vi "State_Machine.vi"(8 "error in (no error)":errorcluster caption="entrée d'erreur (pas d'erreur)", 11 "Get_Voltage en entrée":refnum<class "Enable_Power_Supply.lvclass">) -> (0 "error out":errorcluster caption="sortie d'erreur", 2 "Json_String":string, 3 "Get_Voltage en sortie":refnum<class "Enable_Power_Supply.lvclass">)   [LabVIEW 2020, in "Library Test.lvlib" / "Enable_Power_Supply.lvclass"]
uses:
  Enable_Power_Supply.lvclass
  C:/Users/ngarcin/OneDrive - Altyor/Standard TB/Class/Test/Test (Default)/Test (Default).lvclass
  Instrument/Instrument (Default)/Class Instrument (Default).lvclass
  Enable_Power_Supply.lvclass/Enable_Power_Supply.ctl
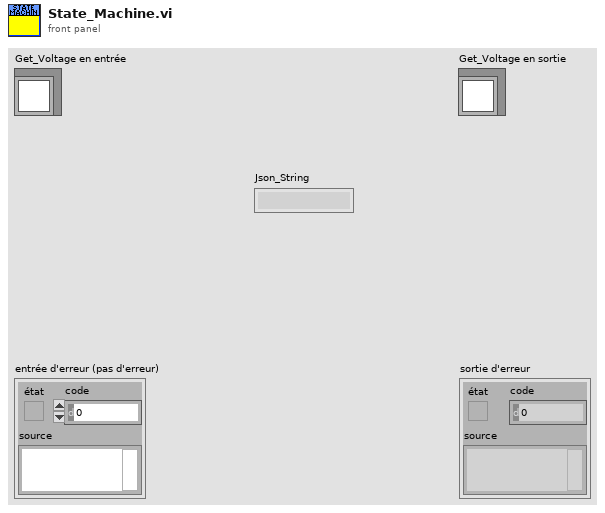
[diagram p1: front panel]
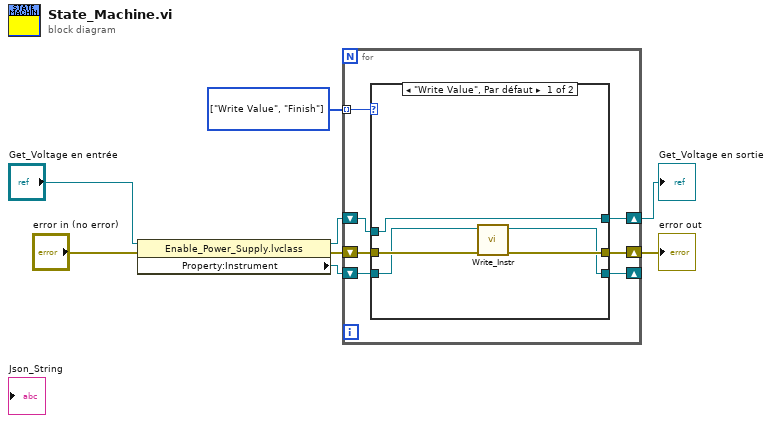
[diagram p0: block diagram]
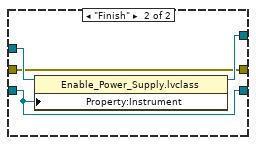
[diagram p2: hidden frame]
diagram:
  w7 = enum16{"Init", "Write Value", "Finish"}[] [enum."Write Value", enum."Finish"] items=["Init", "Write Value", "Finish"]
  n1 = property class="Enable_Power_Supply.lvclass"(reference="Get_Voltage en entrée", error in="error in (no error)") -> (reference out=w5:refnum<class "Enable_Power_Supply.lvclass">, error out=w1:errorcluster, "Property:Instrument"=w6:refnum<class "Class Instrument (Default).lvclass">)
  n2 = for {
    tunnel: w7 -> [w15] mode=indexing
    shift-right: [w13] -> _
    shift-left: w6 -> [w14]
    shift-right: [w11] -> w3
    shift-left: w5 -> [w12]
    shift-right: [w9] -> w4
    shift-left: w1 -> [w10]
    n3 = case shown="\"Write Value\", Par défaut" w15 {
      tunnel: w14 -> [w16 w22]
      tunnel: [w17 w22] -> w13
      tunnel: w12 -> [w20 w24]
      tunnel: [w20 w23] -> w11
      tunnel: w10 -> [w19 w21]
      tunnel: [w18 w21] -> w9
      frame "Write Value", Default {
        n4 = call-dynamic "Write_Instr.vi"("error in (no error)"=w19, "Class Multimeter (Default) en entrée"=w16) -> ("error out"=w18:errorcluster, "Class Multimeter (Default) en sortie"=w17:refnum<class "Class Instrument (Default).lvclass">)  [unwired: 8 in]
      }
      frame "Finish" {
        n5 = property class="Enable_Power_Supply.lvclass"(reference=w24, "Property:Instrument"=w22) -> (reference out=w23:refnum<class "Enable_Power_Supply.lvclass">)  [unwired: 1 in, 1 out]
      }
    }
  }
  "error out" <- w4
  "Get_Voltage en sortie" <- w3
